vi "Equalization.vi"(0 "data in":T1[](array[typedef])=[{"I"=0.0, "Q"=0.0, "overflow"=FALSE}, {"I"=0.0, "Q"=0.0, "overflow"=FALSE}], 9 "input valid":bool, 11 "acq in":refnum<class "niUSRP Rx DSP v2 FPGA.lvclass">) -> (4 "data out":T1[](array[typedef]), 10 "output valid":bool, 14 "ready for input":bool, 15 "acq out":refnum<class "niUSRP Rx DSP v2 FPGA.lvclass">)   [LabVIEW 2025, in "niUSRP Rx DSP v2 FPGA.lvclass"]
uses:
  niUSRP Rx DSP v2 FPGA.lvclass
  <instrlib>/_niInstr/DSP/v1/Shared/Public/IQ Data.ctl
  <instrlib>/_niInstr/DSP Control/Interface/v1/FPGA/Equalization/IQ 18-bit/Equalization Interface (IQ 18-bit).lvclass
  <instrlib>/_niInstr/Basic Elements/v1/FPGA/niInstr Basic Elements v1 FPGA.lvlib
  <instrlib>/_niInstr/DSP/v1/Shared/niInstr DSP v1 Shared.lvlib
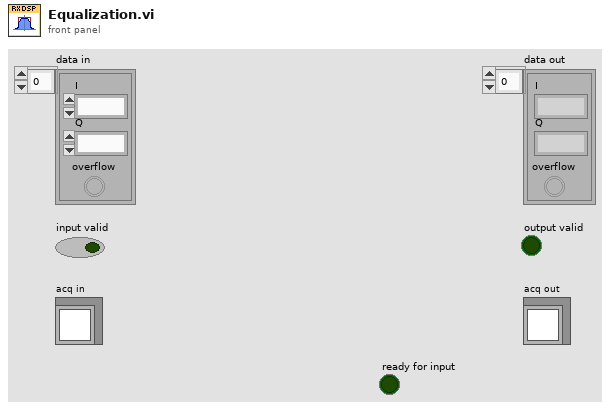
[diagram p1: front panel]
types:
  T1 = typedef "niInstr DSP v1 Shared.lvlib/IQ Data.ctl" = cluster{"I":fxp<+/-,18,1>, "Q":fxp<+/-,18,1>, "overflow":bool}
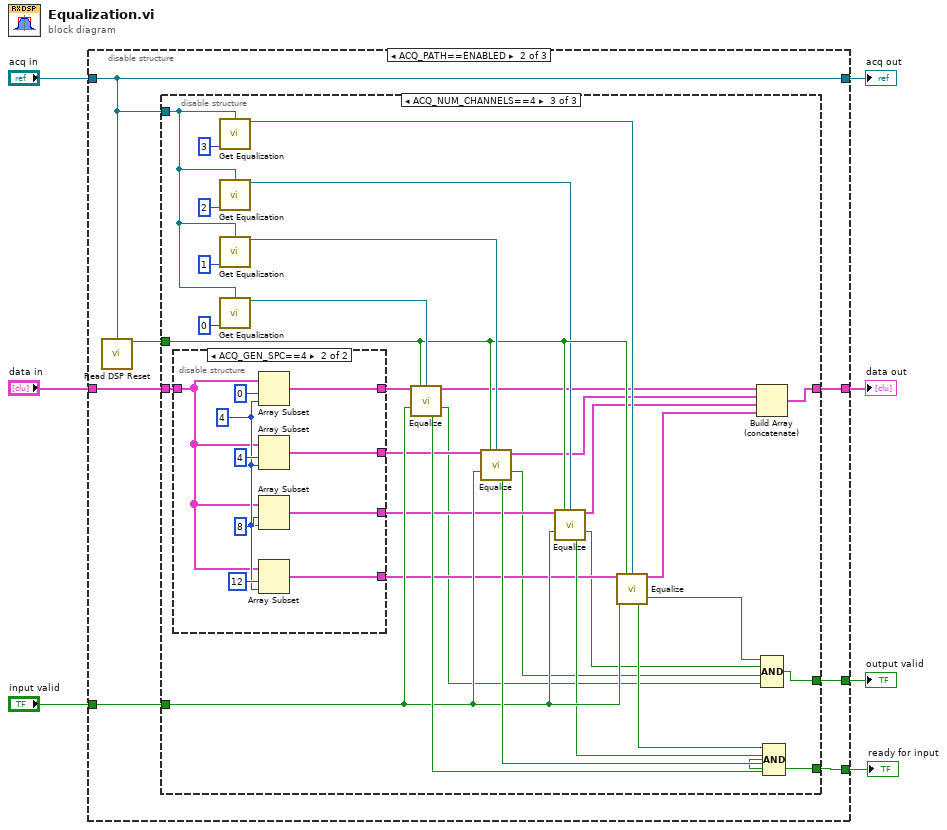
[diagram p0: block diagram]
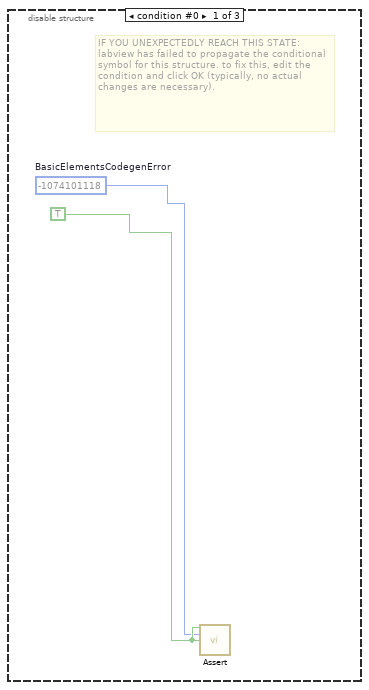
[diagram p2: hidden frame]
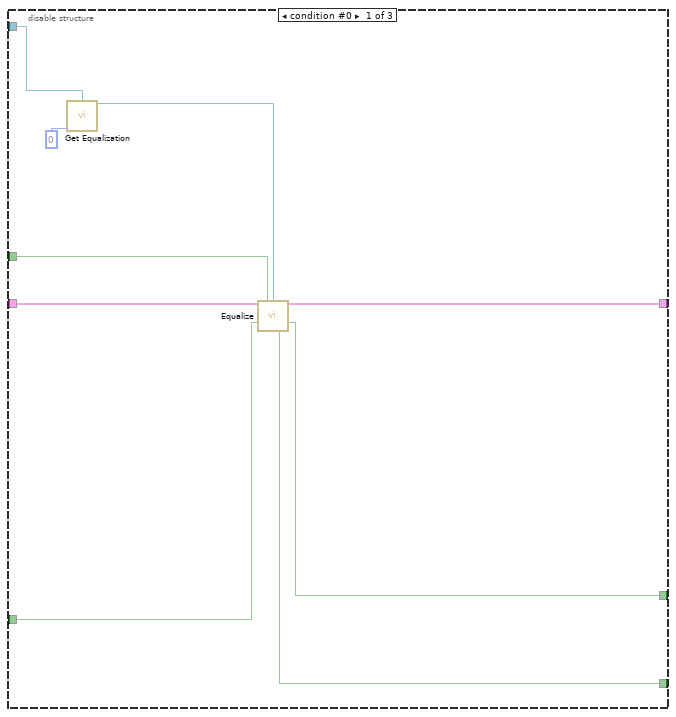
[diagram p3: hidden frame]
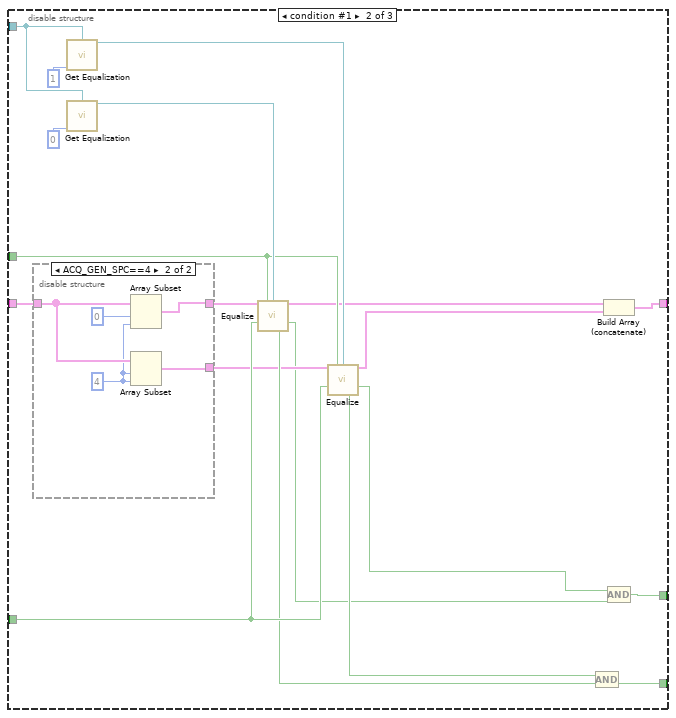
[diagram p4: hidden frame]
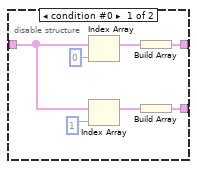
[diagram p5: hidden frame]
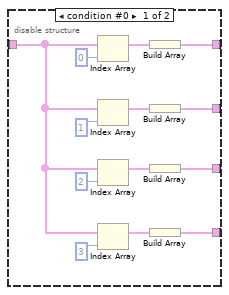
[diagram p6: hidden frame]
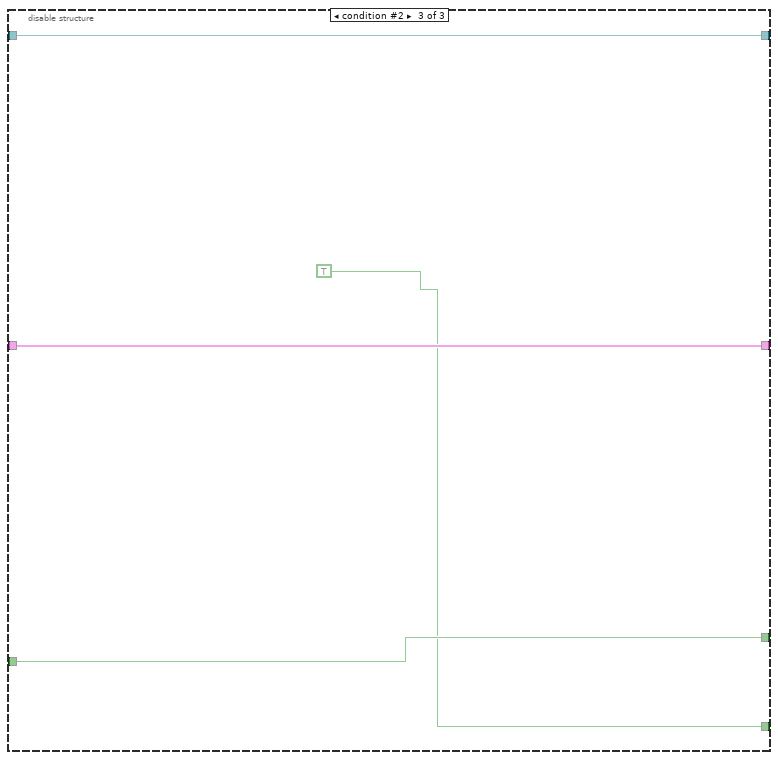
[diagram p7: hidden frame]
diagram:
  n1 = disable-structure shown="ACQ_PATH==ENABLED" {
    disable-tunnel: [_ w16 w113] -> w7
    disable-tunnel: [_ w15 w112] -> w6
    disable-tunnel: "input valid" -> [_ w14 w112]
    disable-tunnel: "data in" -> [_ w11 w113]
    disable-tunnel: "acq in" -> [_ w12 w114]
    disable-tunnel: [_ w12 w114] -> w3
    disable-tunnel: [_ w10 TRUE ("ready for input")] -> w2
    frame condition #0 {
      w9 = TRUE ("assert")
      w8 = -1074101118  # BasicElementsCodegenError
      # "IF YOU UNEXPECTEDLY REACH THIS STATE:\nlabview has failed to propagate the conditional symbol for this structure. to fix this, edit the condition and click OK (typically, no actual changes are necessary)."
      n2 = call <instrlib>:"Assert.vi"("assert"=w9, "error code"=w8, "enable show error"=w9) -> ()  [unwired: 13 in]
    }
    frame condition #1 (active) {
      n3 = call-dynamic "Read DSP Reset.vi"("acq"=w12) -> ("dsp reset"=w13:bool)  [unwired: 14 in]
      n4 = disable-structure shown="ACQ_NUM_CHANNELS==4" {
        disable-tunnel: [w25 w33 w79] -> w16
        disable-tunnel: [w19 w37 w83] -> w15
        disable-tunnel: w14 -> [w20 w38 w72]
        disable-tunnel: w13 -> [w21 w39 w78]
        disable-tunnel: w12 -> [w23 w43 w75]
        disable-tunnel: w11 -> [w17 w32 w69]
        disable-tunnel: [w18 w34 w80] -> w10
        frame condition #0 {
          n5 = call-dynamic "Get Equalization.vi"("acq in"=w23, "ch"=u8 0) -> ("equalization"=w24:refnum<class "Equalization Interface (IQ 18-bit).lvclass">)  [unwired: 13 in]
          n6 = call-dynamic "Equalize.vi"("data in"=w17, "reset"=w21, "equalization"=w24, "input valid"=w20) -> ("data out"=w25:T1[], "output valid"=w19:bool, "ready for input"=w18:bool)  [unwired: 8 in, 1 out]
        }
        frame condition #1 {
          n7 = disable-structure shown="ACQ_GEN_SPC==4" {
            disable-tunnel: w32 -> [w47 w54]
            disable-tunnel: [w46 w55] -> w31
            disable-tunnel: [w45 w53] -> w30
            frame condition #0 {
              n8 = Index Array(array=w47, index=0) -> (element=w51:T1)
              n9 = Index Array(array=w47, index=1) -> (element=w49:T1)
              n10 = Build Array(w51) -> (w46:T1[])
              n11 = Build Array(w49) -> (w45:T1[])
            }
            frame condition #1 (active) {
              w52 = 4 ("length")
              n12 = Array Subset(array=w54, index=0, length=w52) -> (w55:T1[])
              n13 = Array Subset(array=w54, index=w52, length=w52) -> (w53:T1[])
            }
          }
          n14 = call-dynamic "Get Equalization.vi"("acq in"=w43, "ch"=u8 1) -> ("equalization"=w40:refnum<class "Equalization Interface (IQ 18-bit).lvclass">)  [unwired: 13 in]
          n15 = call-dynamic "Get Equalization.vi"("acq in"=w43, "ch"=u8 0) -> ("equalization"=w44:refnum<class "Equalization Interface (IQ 18-bit).lvclass">)  [unwired: 13 in]
          n16 = call-dynamic "Equalize.vi"("data in"=w31, "reset"=w39, "equalization"=w44, "input valid"=w38) -> ("data out"=w29:T1[], "output valid"=w26:bool, "ready for input"=w35:bool)  [unwired: 8 in, 1 out]
          n17 = call-dynamic "Equalize.vi"("data in"=w30, "reset"=w39, "equalization"=w40, "input valid"=w38) -> ("data out"=w28:T1[], "output valid"=w27:bool, "ready for input"=w36:bool)  [unwired: 8 in, 1 out]
          n18 = Compound Arithmetic op=AND(w36, w35) -> (w34:bool)
          n19 = Build Array (concatenate)(w29, w28) -> (w33:T1[])
          n20 = Compound Arithmetic op=AND(w27, w26) -> (w37:bool)
        }
        frame condition #2 (active) {
          n21 = disable-structure shown="ACQ_GEN_SPC==4" {
            disable-tunnel: [w96 w104] -> w68
            disable-tunnel: [w95 w103] -> w67
            disable-tunnel: [w94 w102] -> w66
            disable-tunnel: w69 -> [w89 w105]
            disable-tunnel: [w88 w101] -> w65
            frame condition #0 {
              n22 = Index Array(array=w89, index=0) -> (element=w100:T1)
              n23 = Index Array(array=w89, index=1) -> (element=w98:T1)
              n24 = Index Array(array=w89, index=2) -> (element=w90:T1)
              n25 = Index Array(array=w89, index=3) -> (element=w92:T1)
              n26 = Build Array(w100) -> (w96:T1[])
              n27 = Build Array(w98) -> (w95:T1[])
              n28 = Build Array(w90) -> (w94:T1[])
              n29 = Build Array(w92) -> (w88:T1[])
            }
            frame condition #1 (active) {
              w106 = 4 ("length")
              n30 = Array Subset(array=w105, index=0, length=w106) -> (w104:T1[])
              n31 = Array Subset(array=w105, index=4, length=w106) -> (w103:T1[])
              n32 = Array Subset(array=w105, index=8, length=w106) -> (w102:T1[])
              n33 = Array Subset(array=w105, index=12, length=w106) -> (w101:T1[])
            }
          }
          n34 = call-dynamic "Get Equalization.vi"("acq in"=w75, "ch"=u8 3) -> ("equalization"=w73:refnum<class "Equalization Interface (IQ 18-bit).lvclass">)  [unwired: 13 in]
          n35 = call-dynamic "Get Equalization.vi"("acq in"=w75, "ch"=u8 2) -> ("equalization"=w74:refnum<class "Equalization Interface (IQ 18-bit).lvclass">)  [unwired: 13 in]
          n36 = call-dynamic "Get Equalization.vi"("acq in"=w75, "ch"=u8 1) -> ("equalization"=w84:refnum<class "Equalization Interface (IQ 18-bit).lvclass">)  [unwired: 13 in]
          n37 = call-dynamic "Get Equalization.vi"("acq in"=w75, "ch"=u8 0) -> ("equalization"=w87:refnum<class "Equalization Interface (IQ 18-bit).lvclass">)  [unwired: 13 in]
          n38 = call-dynamic "Equalize.vi"("data in"=w68, "reset"=w78, "equalization"=w87, "input valid"=w72) -> ("data out"=w64:T1[], "output valid"=w57:bool, "ready for input"=w81:bool)  [unwired: 8 in, 1 out]
          n39 = call-dynamic "Equalize.vi"("data in"=w67, "reset"=w78, "equalization"=w84, "input valid"=w72) -> ("data out"=w63:T1[], "output valid"=w58:bool, "ready for input"=w82:bool)  [unwired: 8 in, 1 out]
          n40 = call-dynamic "Equalize.vi"("data in"=w66, "reset"=w78, "equalization"=w74, "input valid"=w72) -> ("data out"=w62:T1[], "output valid"=w59:bool, "ready for input"=w71:bool)  [unwired: 8 in, 1 out]
          n41 = call-dynamic "Equalize.vi"("data in"=w65, "reset"=w78, "equalization"=w73, "input valid"=w72) -> ("data out"=w61:T1[], "output valid"=w60:bool, "ready for input"=w70:bool)  [unwired: 8 in, 1 out]
          n42 = Build Array (concatenate)(w64, w63, w62, w61) -> (w79:T1[])
          n43 = Compound Arithmetic op=AND(w60, w59, w58, w57) -> (w83:bool)
          n44 = Compound Arithmetic op=AND(w70, w71, w82, w81) -> (w80:bool)
        }
      }
    }
    frame condition #2 {
    }
  }
  "data out" <- w7
  "output valid" <- w6
  "ready for input" <- w2
  "acq out" <- w3
